vi "Runtime Si image.vi"(10 "Lamp array":bool[](array[boolean]), 11 "SI camera info":T1={"Observer Name"="", "object name"="", "File name base"="", "Camera Color"="Red", "Exp type tab"="", "Number of Exp"=1, "Exp time"=0, "CCD Readout Speed"=5, "CCD ROI Mode"=10, "Hg(Ar)"=FALSE, "Cu"=FALSE, "Ne"=FALSE, "Bulb"=FALSE, "Ar"=FALSE, "Quartz"=FALSE, "Quartz Percent"=0, "Fe"=FALSE, "Notes"="", "Target Number"="", "DomePercent"=0, "Dome"=FALSE, "Start"=0.0, "Delta"=0.0, "Steps"=0.0, "Custom Roi"={0, 4096, 1, 0, 4096, 1}} {"DomePercent" min=0 step=1; "Quartz Percent" min=0 step=1; "CCD Readout Speed" items=["750 kHz, ATTN 0", "750 kHz, ATTN 2", "344 kHz, ATTN 0", "344 kHz, ATTN 3", "100 kHz, ATTN 2", "100 kHz, ATTN 3"]; "CCD ROI Mode" items=["Imaging, 1x1  "=0, "Imaging, 2x2"=1, "Imaging, 3x3"=2, "Spectroscopic, 1x1"=3, "Spectroscopic, 2x2"=4, "Spectroscopic, 3x3"=5, "MOS, 1x1"=11, "MOS, 2x2"=12, "MOS, 3x3"=13, "Slicer"=6, "Spectroscopic, ZZ Ceti"=14, "Slit Imaging/Alignment"=7, "MOS Imaging/Alignment"=10, "Set user-defined ROI..."=21, "Custom Mode"=9]; "Number of Exp" min=0 step=1; "Exp time" min=0 step=1}) -> (1 "Lamp array 2":bool[](array[boolean]), 3 "time":dbl)   [LabVIEW 2015]
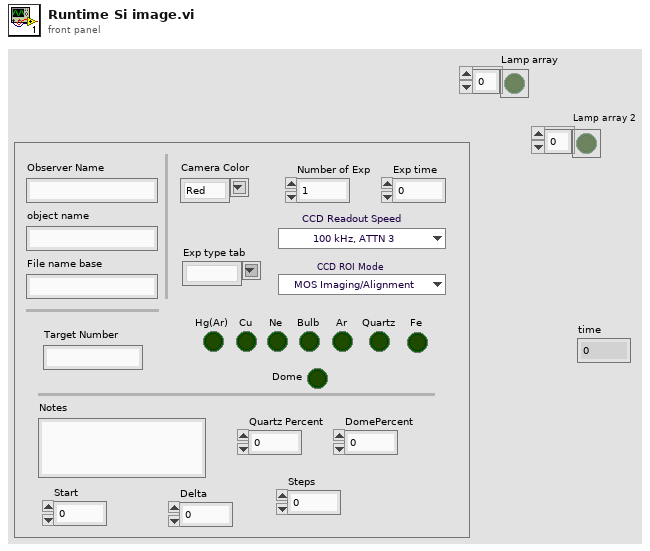
[diagram p1: front panel]
types:
  T1 = cluster{"Observer Name":string, "object name":string, "File name base":string, "Camera Color":string, "Exp type tab":string, "Number of Exp":i32, "Exp time":i32, "CCD Readout Speed":u8, "CCD ROI Mode":u16, "Hg(Ar)":bool, "Cu":bool, "Ne":bool, "Bulb":bool, "Ar":bool, "Quartz":bool, "Quartz Percent":i32, "Fe":bool, "Notes":string, "Target Number":string, "DomePercent":i32, "Dome":bool, "Start":dbl, "Delta":dbl, "Steps":dbl, "Custom Roi":cluster{i32, i32, i32, i32, i32, i32}}
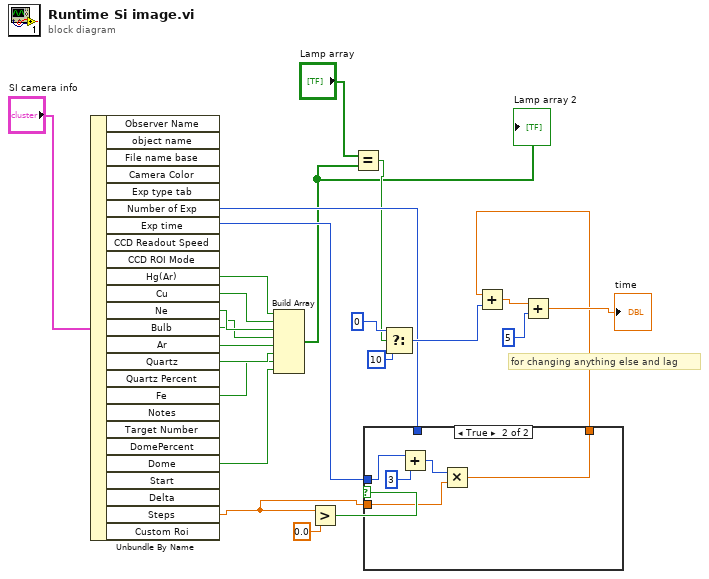
[diagram p0: block diagram]
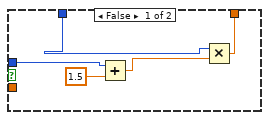
[diagram p2: hidden frame]
diagram:
  # "for changing anything else and lag"
  n1 = Unbundle By Name("SI camera info") -> ("Number of Exp"=w7:i32, "Exp time"=w8:i32, "Hg(Ar)"=w23:bool, "Cu"=w22:bool, "Ne"=w21:bool, "Bulb"=w20:bool, "Ar"=w19:bool, "Quartz"=w18:bool, "Fe"=w17:bool, "Dome"=w16:bool, "Steps"=w5:dbl)  [unwired: 14 out]
  n2 = Build Array(w23, w22, w21, w20, w19, w18, w17, w16) -> (w1:bool[])
  "Lamp array 2" <- w1
  n3 = Greater?(x=w5, y=0.0) -> (0:w9:bool)
  n4 = Equal?(x="Lamp array", y=w1) -> (x = y?=w2:bool)
  n5 = case shown="True" w9 {
    tunnel: w8 -> [w27 w34]
    tunnel: w7 -> [w26 _]
    tunnel: [w25 w30] -> w6
    tunnel: w5 -> [_ w31]
    frame False {
      n6 = Add(x=w27, y=1.5) -> (x+y=w29:dbl)
      n7 = Multiply(x=w26, y=w29) -> (x*y=w25:dbl)
    }
    frame True {
      n8 = Add(x=w34, y=3) -> (x+y=w32:i32)
      n9 = Multiply(x=w32, y=w31) -> (x*y=w30:dbl)
    }
  }
  n10 = Select(t=0, s=w2, f=10) -> (s? t:f=w14:i32)
  n11 = Add(x=w6, y=w14) -> (x+y=w13:dbl)
  n12 = Add(x=w13, y=5) -> (x+y=→"time":dbl)
